vi "PixelCombi.vi"(8 "error in":errorcluster, 10 "quantity":i32=4, 11 "array":i32[](array[numeric])) -> (0 "error out":errorcluster, 1 "Channels":i32[](array[numeric]), 2 "Combination Array":i16[](array[numeric]))   [LabVIEW 2009]
doc: "This VI generates an array containing all numbers between 0-256 that has 4 logical ones in its binary respresentation."
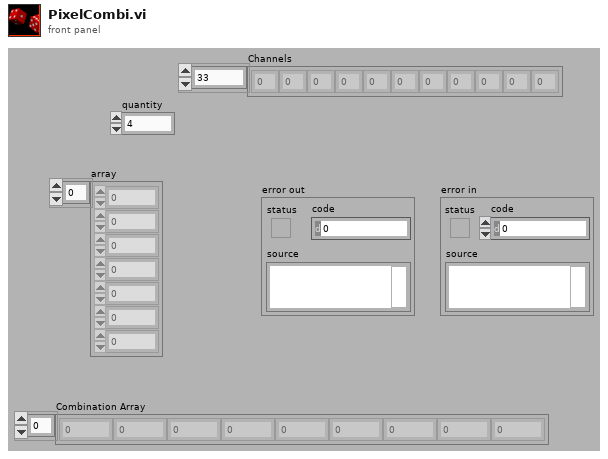
[diagram p1: front panel]
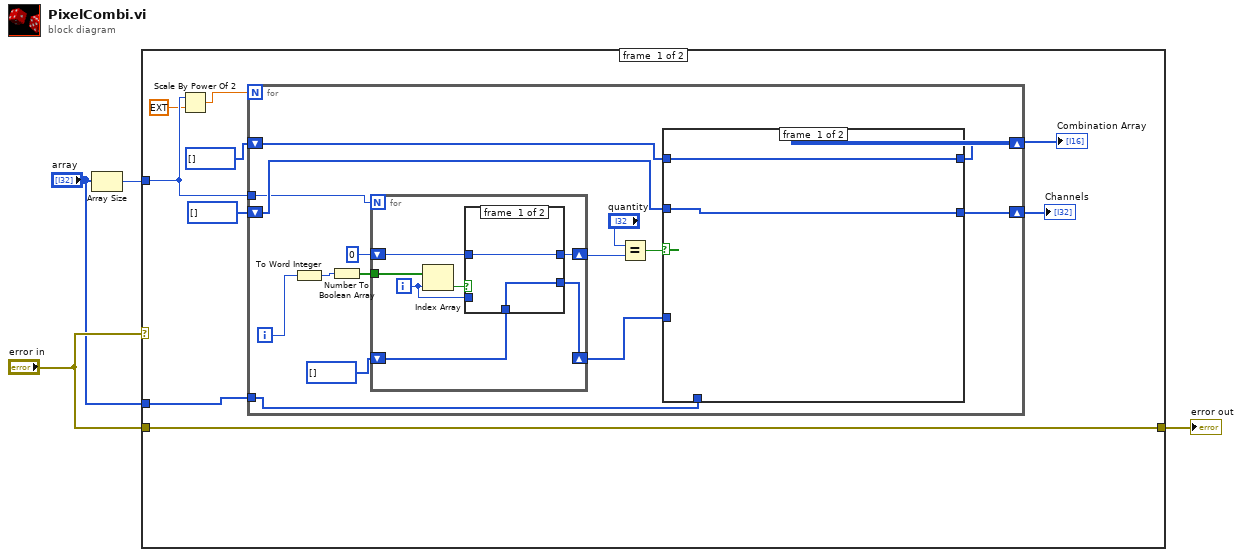
[diagram p0: block diagram]
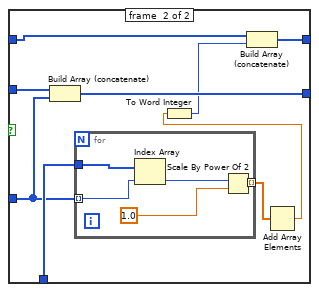
[diagram p2: hidden frame]
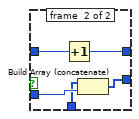
[diagram p3: hidden frame]
diagram:
  n1 = Array Size(array="array") -> (size(s)=w2:i32)
  n2 = case shown="No Error" "error in" {
    tunnel: "error in" -> [w11 w59]
    tunnel: [w11 w59] -> w4
    tunnel: w2 -> [w8 _]
    tunnel: "array" -> [w5 _]
    frame #0 {
      n3 = Scale By Power Of 2(n=w8, x=ext 1.0) -> (x*2^n=w6:ext)
      n4 = for {
        N: w6 -> [_]
        shift-right: [w21] -> w12
        shift-left: i16[] [] -> [w20]
        shift-right: [w18] -> w9
        shift-left: i32[] [] -> [w17]
        tunnel: w8 -> [w16]
        tunnel: w5 -> [w14]
        i -> [w28]
        n5 = To Word Integer(number=w28) -> (16bit integer=w22:i16)
        n6 = Number To Boolean Array(number=w22) -> (Boolean array=w27:bool[])
        n7 = for {
          N: w16 -> [_]
          tunnel: w27 -> [w51]
          shift-right: [w48] -> w25
          shift-left: 0 -> [w49]
          shift-right: [w46] -> w15
          shift-left: i32[] [] -> [w45]
          i -> [w47]
          n8 = Index Array(array=w51, index=w47) -> (element=w50:bool)
          n9 = case shown="True" w50 {
            tunnel: w49 -> [w53 w58]
            tunnel: [w53 w57] -> w48
            tunnel: w47 -> [_ w56]
            tunnel: [w52 w55] -> w46
            tunnel: w45 -> [w52 w54]
            frame #0 {
            }
            frame #1 {
              n10 = Increment(x=w58) -> (x+1=w57:i32)
              n11 = Build Array (concatenate)(w54, w56) -> (w55:i32[])
            }
          }
        }
        n12 = Equal?(x="quantity", y=w25) -> (x = y?=w23:bool)
        n13 = case shown="True" w23 {
          tunnel: [w30 w39] -> w21
          tunnel: w20 -> [w30 w38]
          tunnel: w14 -> [_ w34]
          tunnel: [w29 w37] -> w18
          tunnel: w17 -> [w29 w36]
          tunnel: w15 -> [_ w33]
          frame #0 {
          }
          frame #1 {
            n14 = Build Array (concatenate)(w36, w33) -> (w37:i32[])
            n15 = for {
              tunnel: w34 -> [w44]
              tunnel: w33 -> [w43] mode=indexing
              tunnel: [w41] -> w35 mode=indexing
              n16 = Index Array(array=w44, index=w43) -> (element=w40:i32)
              n17 = Scale By Power Of 2(n=w40, x=1.0) -> (x*2^n=w41:dbl)
            }
            n18 = Add Array Elements(numeric array=w35) -> (sum=w32:dbl)
            n19 = To Word Integer(number=w32) -> (16bit integer=w31:i16)
            n20 = Build Array (concatenate)(w38, w31) -> (w39:i16[])
          }
        }
      }
      "Combination Array" <- w12
      "Channels" <- w9
    }
    frame #1 {
    }
  }
  "error out" <- w4
